vi "CreatingName_UsuallyInstrument.vi"(2 "error in (no error)":errorcluster) -> (0 "error in (no error) 2":errorcluster, 1 "Output Name":string)   [LabVIEW 2019]
panel:
  in  "Name":string
  in  "Confirm Name":bool
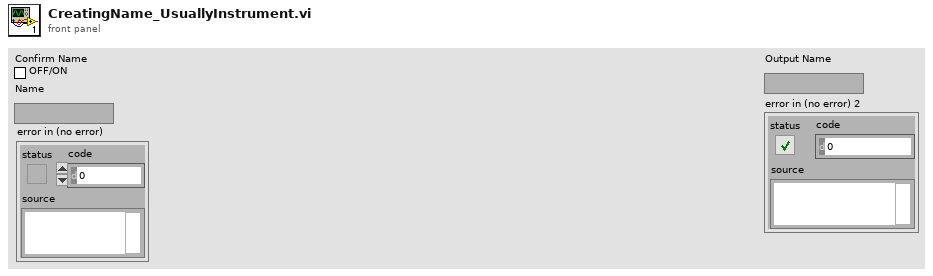
[diagram p1: front panel]
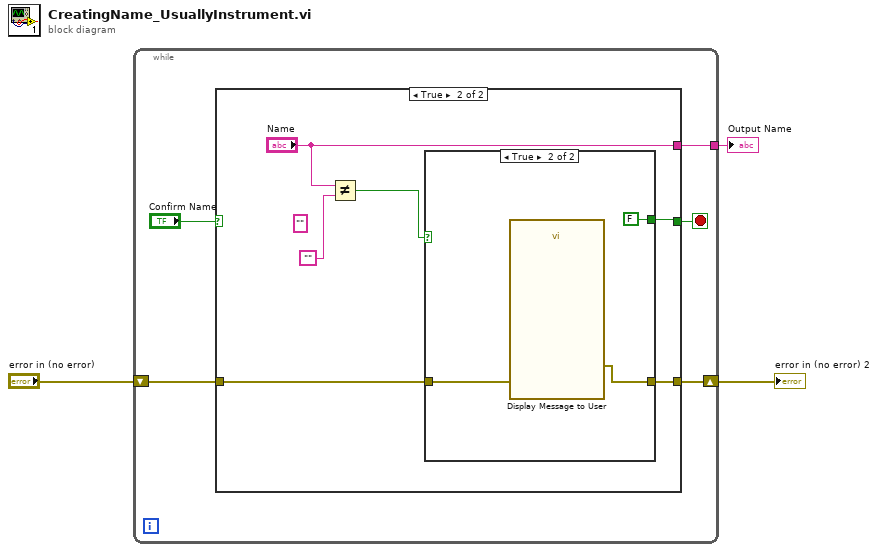
[diagram p0: block diagram]
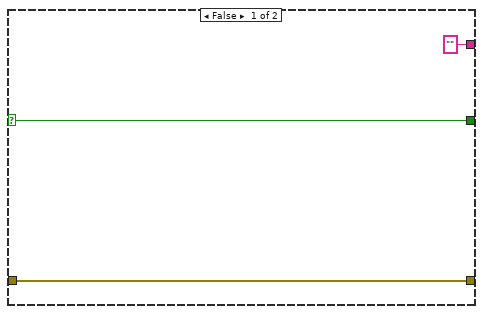
[diagram p2: hidden frame]
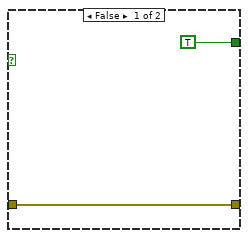
[diagram p3: hidden frame]
diagram:
  n1 = while {
    shift-right: [w6] -> w1
    shift-left: "error in (no error)" -> [w7]
    tunnel: [w5] -> w2
    stop <- w4 stop-if-true
    n2 = case shown="True" "Confirm Name" {
      selector: "Confirm Name" -> [w9 _]
      tunnel: w7 -> [w11 w15]
      tunnel: [w11 w14] -> w6
      tunnel: ["" ("Name") "Name"] -> w5
      tunnel: [w9 w12] -> w4
      frame False {
      }
      frame True {
        (unwired) ""
        n3 = Not Equal?(x="Name", y="") -> (x != y?=w16:bool)
        n4 = case shown="True" w16 {
          tunnel: w15 -> [w19 w22]
          tunnel: [w19 w21] -> w14
          tunnel: [TRUE FALSE] -> w12
          frame False {
          }
          frame True {
            n5 = call "Display Message to User"("error in (no error)"=w22) -> ("error out"=w21:errorcluster)  [unwired: 9 in, 1 out]
          }
        }
      }
    }
  }
  "Output Name" <- w2
  "error in (no error) 2" <- w1
